vi "ChooseResultsFile.vi"(8 "error in (no error)":errorcluster, 11 "ResultsViewer in":refnum<class "ResultsViewer.lvclass">) -> (0 "error out":errorcluster, 2 "Cancelled?":bool, 3 "ResultsViewer out":refnum<class "ResultsViewer.lvclass">)   [LabVIEW 2019, in "ResultsViewer.lvlib" / "ResultsViewer.lvclass"]
uses:
  ResultsViewer.lvclass
  ResultsViewer.lvclass/ResultsViewer.ctl
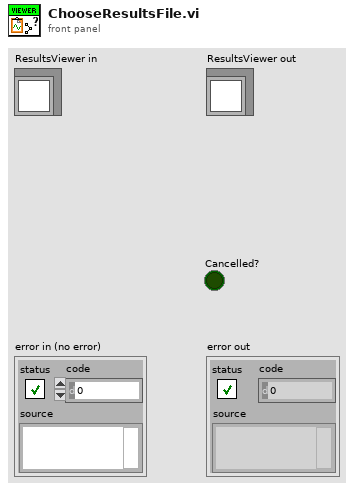
[diagram p1: front panel]
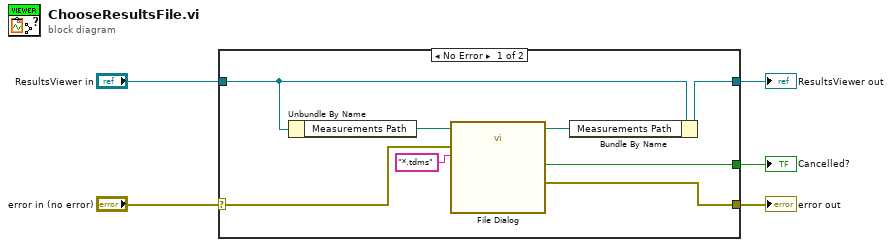
[diagram p0: block diagram]
diagram:
  n1 = case shown="No Error" "error in (no error)" {
    selector: "error in (no error)" -> [w11 w15]
    tunnel: [w10 w15] -> w4
    tunnel: [w8 w14] -> w2
    tunnel: "ResultsViewer in" -> [w13 w14]
    tunnel: [w9 _] -> w1
    frame No Error {
      n2 = Unbundle By Name(w13) -> ("Measurements Path"=w7:path)
      n3 = call "File Dialog"("start path"=w7, "error in"=w11, "pattern (all files)"="*.tdms") -> ("selected path"=w6:path, "cancelled"=w9:bool, "error out"=w10:errorcluster)  [unwired: 9 in, 1 out]
      n4 = Bundle By Name(cluster=w13, "Measurements Path"=w6) -> (w8:refnum<class "ResultsViewer.lvclass">)
    }
    frame Error {
    }
  }
  "error out" <- w4
  "ResultsViewer out" <- w2
  "Cancelled?" <- w1
